vi "BuildFileText.vi"(11 "Code":string) -> (2 "to send":string, 3 "commands":string[](array[string]))   [LabVIEW 2022 SP3]
uses:
  <vilib>/Utility/error.llb/Trim Whitespace One-Sided.vi
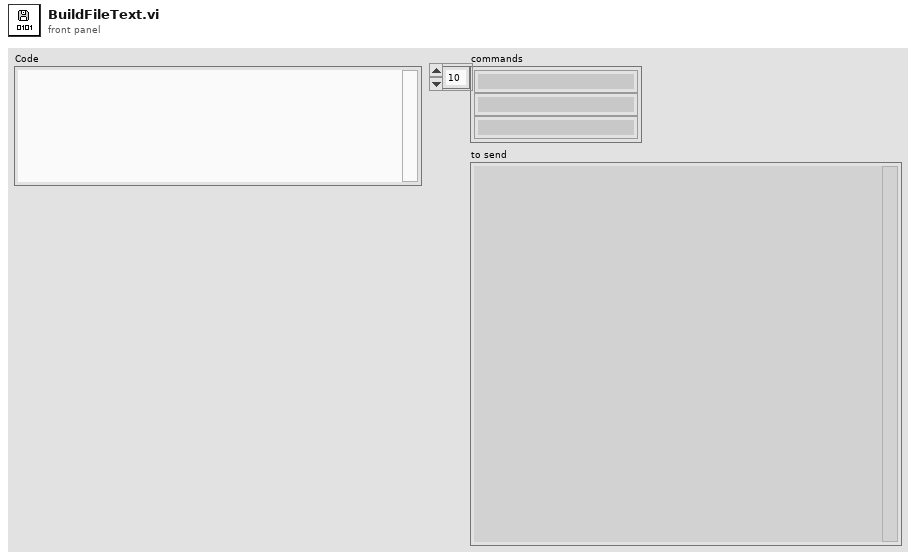
[diagram p1: front panel]
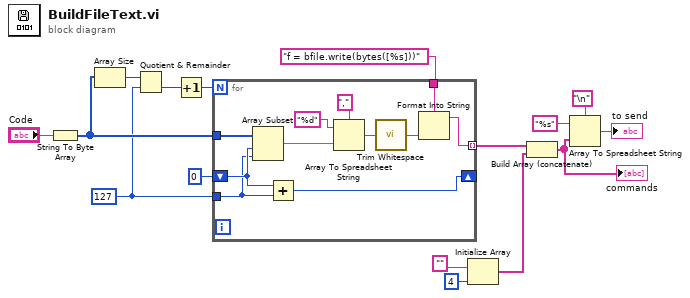
[diagram p0: block diagram]
diagram:
  w5 = 127 ("length (rest)")
  n1 = String To Byte Array(string="Code") -> (unsigned byte array=w14:u8[])
  n2 = Array Size(array=w14) -> (size(s)=w7:i32)
  n3 = Quotient & Remainder(x=w7, y=w5) -> (floor(x/y)=w8:i32)  [unwired: 1 out]
  n4 = Increment(x=w8) -> (x+1=w15:i32)
  n5 = for {
    N: w15 -> [_]
    shift-right: [w26] -> _
    shift-left: 0 -> [w27]
    tunnel: w5 -> [w25]
    tunnel: w14 -> [w24]
    tunnel: [w19] -> w13 mode=indexing
    tunnel: "f = bfile.write(bytes([%s]))" -> [w17]
    n6 = Array Subset(array=w24, index=w27, length=w25) -> (w20:u8[])
    n7 = Add(x=w27, y=w25) -> (x+y=w26:i32)
    n8 = Array To Spreadsheet String(delimiter (Tab)=",", array=w20, 3:"%d" ("format string")) -> (spreadsheet string=w21:string)
    n9 = call <vilib>:"Trim Whitespace.vi"("string"=w21) -> ("trimmed string"=w18:string)  [unwired: 1 in]
    n10 = Format Into String(format string=w17, w18) -> (resulting string=w19:string)  [unwired: 2 in, 1 out]
  }
  n11 = Initialize Array("" ("delimiter (Tab)"), 4 ("dimension size")) -> (w2:string[])
  n12 = Build Array (concatenate)(w13, w2) -> (w9:string[])
  "commands" <- w9
  n13 = Array To Spreadsheet String(delimiter (Tab)="\n", array=w9, 3:"%s" ("format string")) -> (spreadsheet string=→"to send":string)
